vi "setFPGA.vi"(10 "FPGA":refnum<class "FPGA.lvclass">, 11 "ModbusSubnetCTxDataFIFO in":refnum<class "ModbusSubnetCTxDataFIFO.lvclass">) -> (3 "ModbusSubnetCTxDataFIFO out":refnum<class "ModbusSubnetCTxDataFIFO.lvclass">)   [LabVIEW 2016, in "ModbusSubnetCTxDataFIFO.lvclass"]
uses:
  ModbusSubnetCTxDataFIFO.lvclass
  FPGA/FPGA.lvclass
  ModbusSubnetCTxDataFIFO.lvclass/ModbusSubnetCTxDataFIFO.ctl
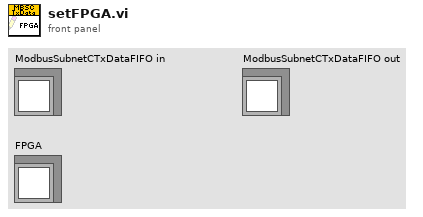
[diagram p1: front panel]
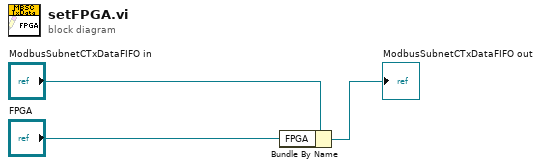
[diagram p0: block diagram]
diagram:
  n1 = Bundle By Name(cluster="ModbusSubnetCTxDataFIFO in", "FPGA"="FPGA") -> (→"ModbusSubnetCTxDataFIFO out":refnum<class "ModbusSubnetCTxDataFIFO.lvclass">)
